vi "Cal RowNum(SubVI) - rgb.vi"(9 "Width":u16, 10 "preRow":u16, 11 "preCol":u16) -> (2 "curRow":u16)   [LabVIEW 2016]
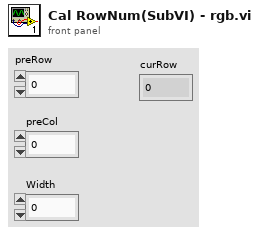
[diagram p1: front panel]
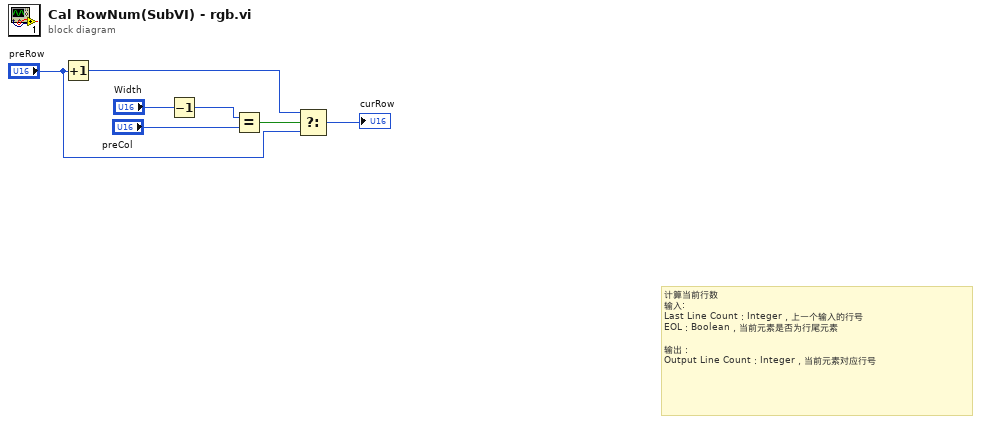
[diagram p0: block diagram]
diagram:
  # "计算当前行数\n输入:\nLast Line Count：Integer，上一个输入的行号\nEOL：Boolean，当前元素是否为行尾元素\n\n输出：\nOutput Line Count：Integer，当前元素对应行号"
  n1 = Increment(x="preRow") -> (x+1=w3:u16)
  n2 = Decrement(x="Width") -> (x-1=w6:u16)
  n3 = Equal?(x=w6, y="preCol") -> (x = y?=w4:bool)
  n4 = Select(t=w3, s=w4, f="preRow") -> (s? t:f=→"curRow":u16)
